vi "Read Message Box.vi"(9 "Downloader in":refnum<class "Downloader.lvclass">) -> (3 "Downloader out":refnum<class "Downloader.lvclass">, 4 "Message Box":refnum<class "MessageBox.lvclass">)   [LabVIEW 2014, in "Downloader.lvclass"]
uses:
  Downloader.lvclass
  MessageBox/MessageBox.lvclass
  Downloader.lvclass/Downloader.ctl
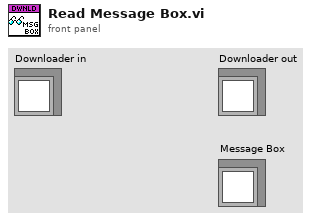
[diagram p1: front panel]
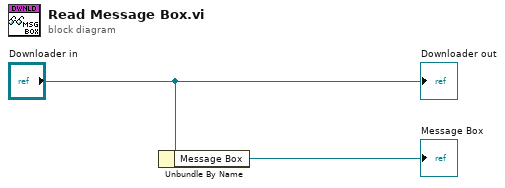
[diagram p0: block diagram]
diagram:
  n1 = Unbundle By Name("Downloader in") -> ("Message Box"=→"Message Box":refnum<class "MessageBox.lvclass">)
  "Downloader out" <- "Downloader in"
